vi "Register Callbacks.vi"(8 "error in (no error)":errorcluster, 11 "Single Node Browser":T1) -> (0 "error out":errorcluster, 2 "Callbacks":T2, 3 "Single Node Browser dup":T1)   [LabVIEW 2020, in "NI_VS UI Single Node Browser.lvlib"]
uses:
  <vilib>/NI VeriStand/UI Controls/Single Node Browser/NI_VS UI Single Node Browser.lvlib
  <vilib>/NI VeriStand/UI Controls/Single Node Browser/Single Node Browser Ref.ctl
  NationalInstruments.VeriStand.SystemStorageUI
  <vilib>/NI VeriStand/UI Controls/Single Node Browser/Callback Type.ctl
  <vilib>/NI VeriStand/UI Controls/Single Node Browser/Net Event Data.ctl
  <vilib>/NI VeriStand/UI Controls/Single Node Browser/Net Event.ctl
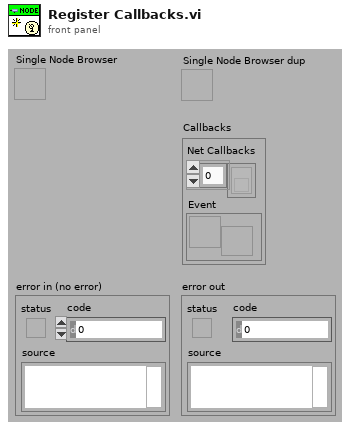
[diagram p1: front panel]
types:
  T1 = typedef "NI_VS UI Single Node Browser.lvlib/Single Node Browser Ref.ctl" = refnum<k24>
  T2 = typedef "NI_VS UI Single Node Browser.lvlib/Callback Type.ctl" = cluster{"Net Callbacks":refnum<k27>[], "Event":refnum<user-event>}
  T3 = typedef "NI_VS UI Single Node Browser.lvlib/Net Event Data.ctl" = cluster{"Event":T4, "Data":variant}
  T4 = typedef "NI_VS UI Single Node Browser.lvlib/Net Event.ctl" = enum16{"SelectedItem"}
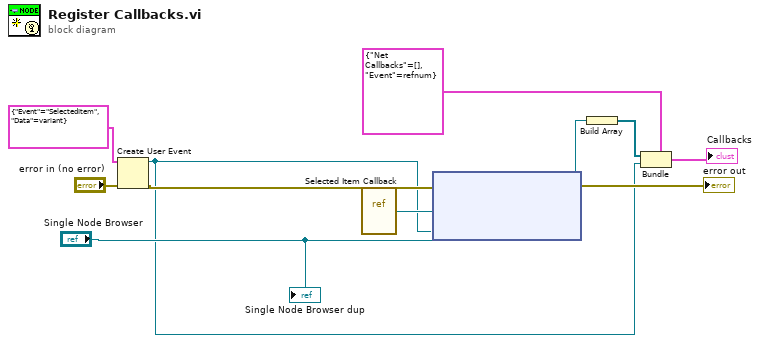
[diagram p0: block diagram]
diagram:
  n1 = Create User Event(user event datatype=T3 {"Event"=enum."SelectedItem", "Data"=variant} ("Net Event Data"), error in="error in (no error)") -> (user event=w1:refnum<user-event>, error out=w6:errorcluster)
  n2 = vi-ref <vilib>:"Selected Item Callback.vi"() -> ("vi reference"=w9:refnum<vi>)
  n3 = node(w6, "Single Node Browser", w9, w1) -> (w7:refnum<k27>, →"error out":errorcluster)  [unwired: 1 in]
  n4 = Build Array(w7) -> (w5:refnum<k27>[])
  n5 = Bundle(cluster=T2 {"Net Callbacks"=[], "Event"=refnum} ("Callback"), "Net Callbacks"=w5, "Event"=w1) -> (→"Callbacks":T2)
  "Single Node Browser dup" <- "Single Node Browser"
